vi "generic.vi"(5 "send":bool=TRUE caption="Send", 7 "override":bool, 8 "error in (no error)":errorcluster, 9 "generic settings":T1={"generic cmd"="", "upper_limit"=5.0, "lower limit"=0.05, "format"="%#.8g"} {"upper_limit" format="%#_13g"}, 10 "Value":dbl, 11 "VISA IN":refnum<visa-resource-name>) -> (0 "error out":errorcluster, 1 "In Range?":bool, 2 "value out":dbl=0.05)   [LabVIEW 2017]
uses:
  tools/core/generic_config.ctl
  tools/tools.lvlib
panel:
  out "command string":string
  in  "VISA (default)":refnum<visa-resource-name>
  # "Send a general command to an instrument, e.g.,\n\n    SOUR1:FUNC:PULS:PER <value>"
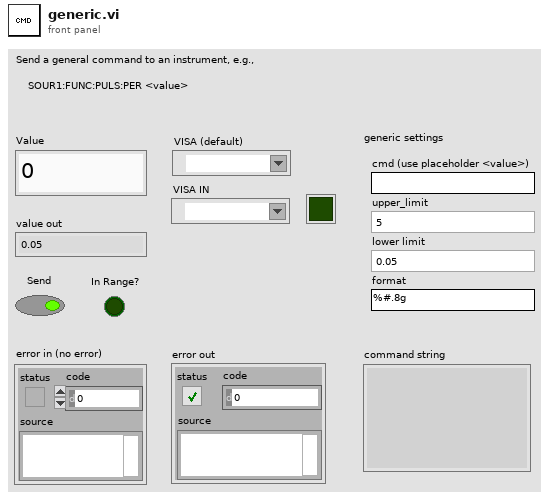
[diagram p1: front panel]
types:
  T1 = typedef "tools.lvlib/generic_config.ctl" = cluster{"generic cmd":string, "upper_limit":dbl, "lower limit":dbl, "format":string}
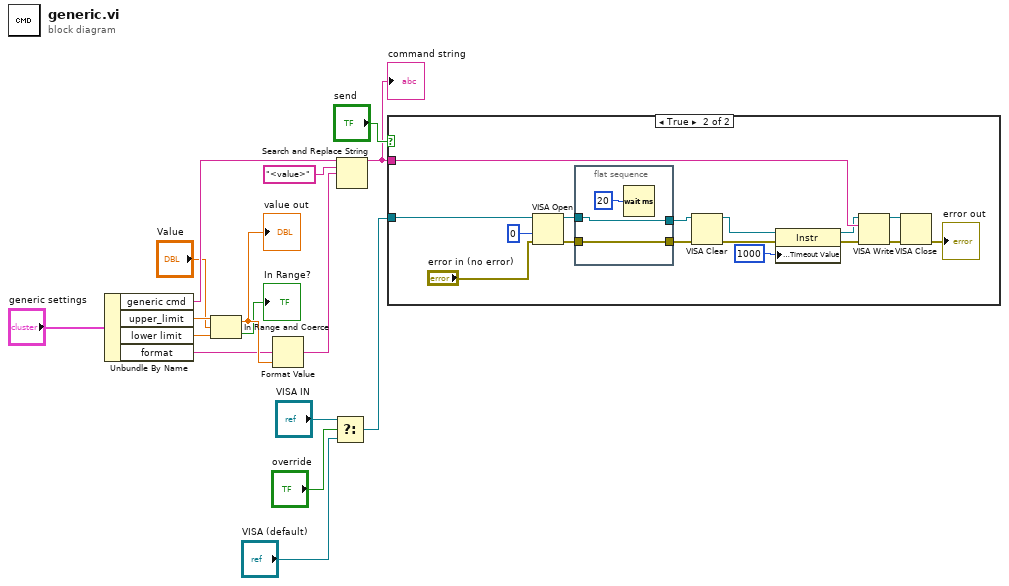
[diagram p0: block diagram]
diagram:
  n1 = Unbundle By Name("generic settings") -> ("generic cmd"=w9:string, "upper_limit"=w8:dbl, "lower limit"=w7:dbl, "format"=w6:string)
  n2 = In Range and Coerce(upper limit=w8, x="Value", lower limit=w7) -> (coerced(x)=w15:dbl, In Range?=→"In Range?":bool)
  "value out" <- w15
  n3 = Format Value(format string=w6, value (0)=w15) -> (output string=w12:string)  [unwired: 1 in]
  n4 = Select(t="VISA IN", s="override", f="VISA (default)") -> (s? t:f=w1:refnum<visa-resource-name>)
  n5 = Search and Replace String(input string=w9, search string="<value>", replace string=w12) -> (result string=w11:string)  [unwired: 5 in, 3 out]
  "command string" <- w11
  n6 = case shown="True" "send" {
    tunnel: w11 -> [_ w29]
    tunnel: w1 -> [_ w21]
    frame False {
    }
    frame True {
      n7 = VISA Open(access mode=u32 0, error in (no error)="error in (no error)", VISA resource name=w21) -> (VISA resource name=w17:refnum<visa-resource-name>, error out=w19:errorcluster)  [unwired: 2 out]
      n8 = flat-sequence {
        tunnel: [w35] -> w20
        tunnel: w19 -> [w35]
        tunnel: [w34] -> w18
        tunnel: w17 -> [w34]
        frame #0 {
          n9 = Wait (ms)(milliseconds to wait=u32 20) -> ()  [unwired: 1 out]
        }
      }
      n10 = VISA Clear(VISA resource name=w18, error in (no error)=w20) -> (VISA resource name out=w27:refnum<visa-resource-name>, error out=w28:errorcluster)
      n11 = property class="Instr"(reference=w27, error in=w28, "General Settings:Timeout Value"=u32 1000) -> (reference out=w23:refnum<visa-resource-name>, error out=w25:errorcluster)
      n12 = VISA Write(VISA resource name=w23, write buffer=w29, error in (no error)=w25) -> (VISA resource name out=w22:refnum<visa-resource-name>, error out=w24:errorcluster)  [unwired: 1 out]
      n13 = VISA Close(VISA resource name=w22, error in (no error)=w24) -> (error out=→"error out":errorcluster)
    }
  }
